vi "Col_Velocity(Subvi).vi"(8 "Fs":dbl=110000.0 format="%#_13g", 9 "거리":dbl format="%#_13g", 10 "Station_index_2":i32, 11 "Station_index_1":i32) -> (0 "Averange_SoundSpeed":dbl, 2 "Water_Velocity":dbl)   [LabVIEW 2024]
panel:
  out "원소":string
  out "출력 배열":string[](array[string])
  out "부분배열 2":string[][](array[string])
  in  "유속 데이터 흐름표_10분":i32(listbox)=-1
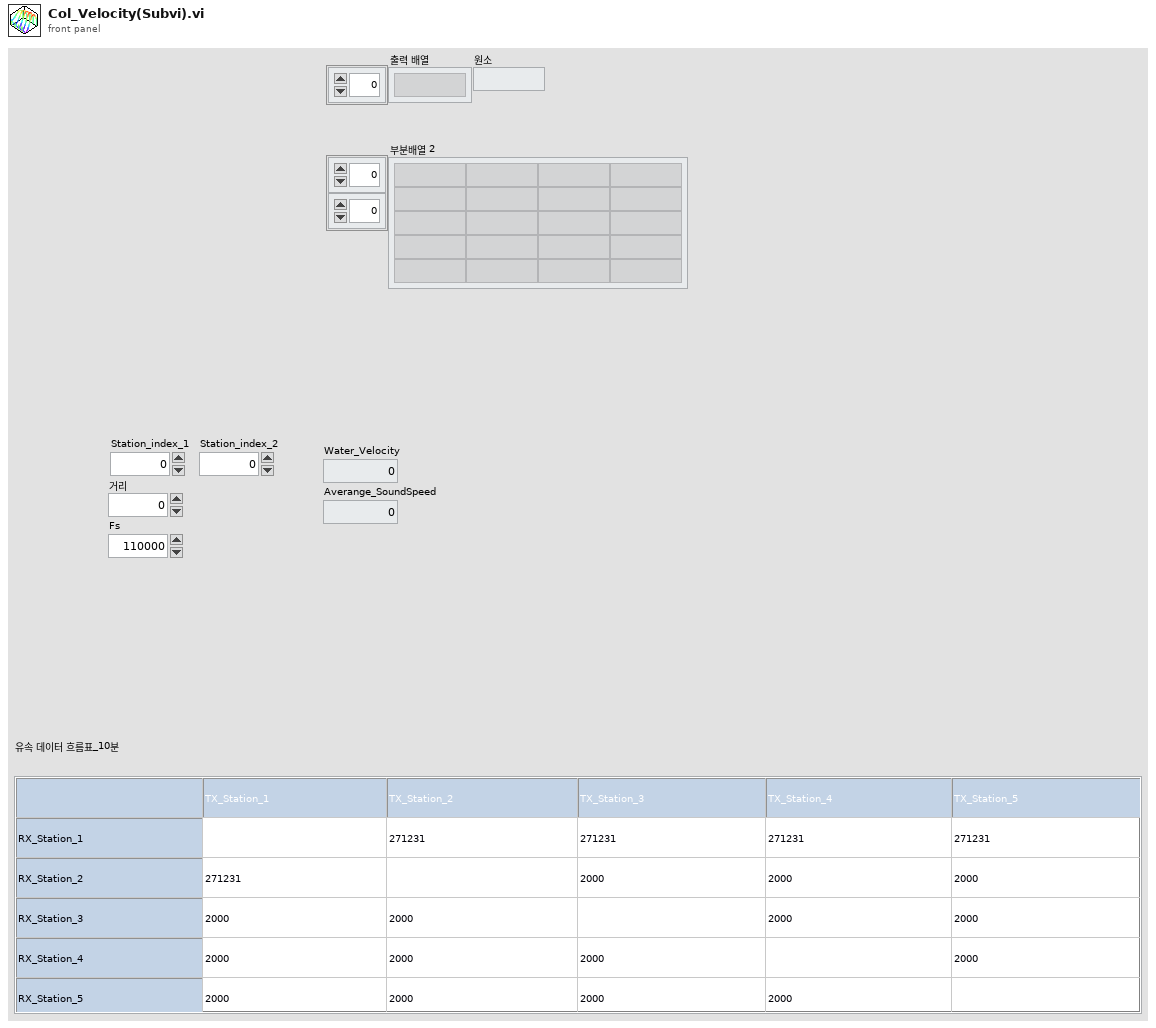
[diagram p1: front panel]
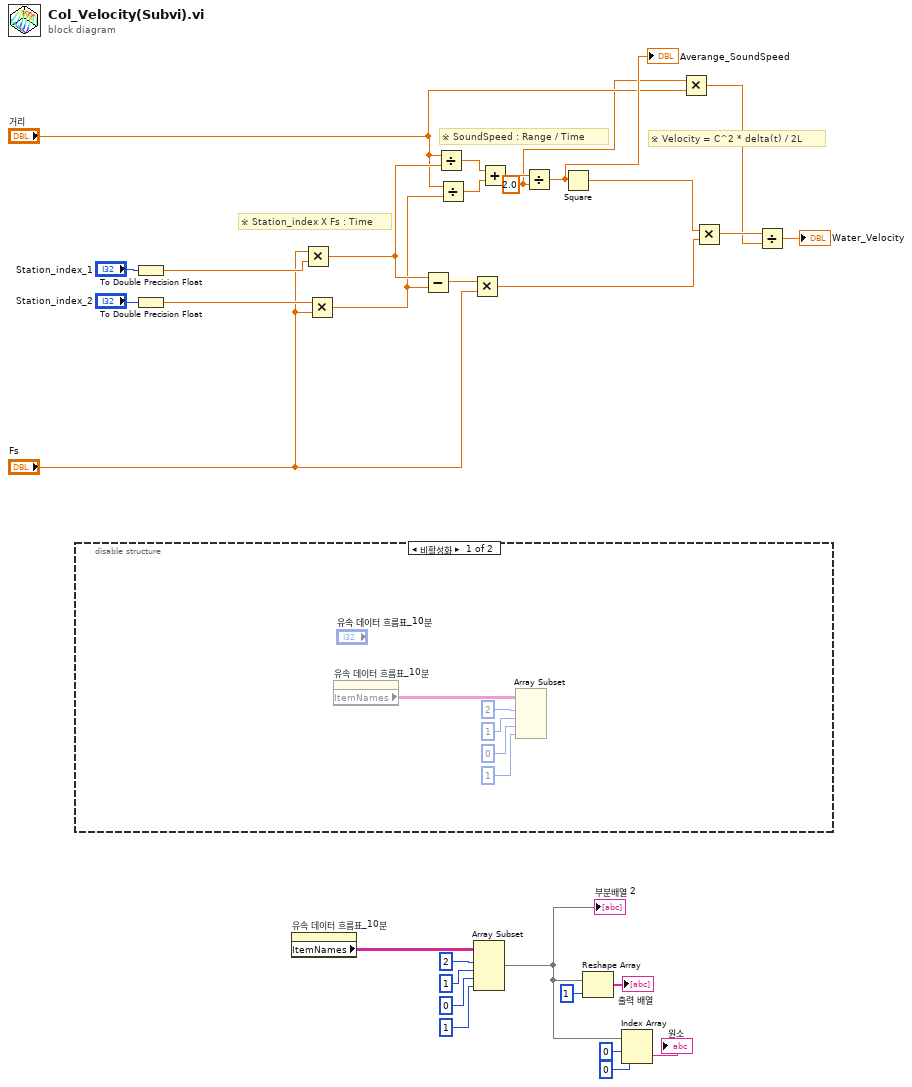
[diagram p0: block diagram]
diagram:
  w13 = 2.0 ("y")
  # "※ Velocity = C^2 * delta(t) / 2L"
  # "※ SoundSpeed : Range / Time"
  # "※ Station_index X Fs : Time"
  n1 = disable-structure shown="비활성화" {
    frame Disabled {
      n2 = property on="유속 데이터 흐름표_10분" class="MCListbox (엄격한)"() -> ("ItemNames"=w35:string[][])  [unwired: 2 in, 2 out]
      n3 = Array Subset(array=w35, index (row)=2 ("인덱스"), length (row)=1 ("길이"), index (col)=0 ("인덱스"), length (col)=1 ("길이")) -> ()  [unwired: 1 out]
    }
    frame Enabled {
    }
  }
  n4 = To Double Precision Float(number="Station_index_1") -> (double precision float=w28:dbl)
  n5 = To Double Precision Float(number="Station_index_2") -> (double precision float=w27:dbl)
  n6 = property on="유속 데이터 흐름표_10분" class="MCListbox (엄격한)"() -> ("ItemNames"=w7:string[][])  [unwired: 2 in, 2 out]
  n7 = Multiply(x="Fs", y=w28) -> (x*y=w24:dbl)
  n8 = Multiply(x=w27, y="Fs") -> (x*y=w23:dbl)
  n9 = Subtract(x=w24, y=w23) -> (x-y=w26:dbl)
  n10 = Divide(x="거리", y=w24) -> (x/y=w22:dbl)
  n11 = Divide(x="거리", y=w23) -> (x/y=w21:dbl)
  n12 = Multiply ("곱하기")(x=w26, y="Fs") -> (x*y=w17:dbl)
  n13 = Array Subset(array=w7, index (row)=2 ("인덱스"), length (row)=1 ("길이"), index (col)=0 ("인덱스"), length (col)=1 ("길이")) -> (w3:string[][])
  "부분배열 2" <- w3
  n14 = Add(x=w22, y=w21) -> (x+y=w20:dbl)
  n15 = Divide(x=w20, y=w13) -> (x/y=w19:dbl)
  "Averange_SoundSpeed" <- w19
  n16 = Square(x=w19) -> (x^2=w18:dbl)
  n17 = Reshape Array(w3, 1 ("차원 크기")) -> (→"출력 배열":string[])
  n18 = Index Array(array=w3, index (row)=0 ("인덱스"), index (col)=0 ("비활성화된 인덱스 (열)")) -> (element=→"원소":string)
  n19 = Multiply(x=w13, y="거리") -> (x*y=w15:dbl)
  n20 = Multiply(x=w18, y=w17) -> (x*y=w16:dbl)
  n21 = Divide(x=w16, y=w15) -> (x/y=→"Water_Velocity":dbl)
